vi "Change.vi"(6 "OldVal":variant, 8 "error in (no error)":errorcluster, 9 "NewVal":variant, 10 "Control Index":i32=-1, 11 "UndoObject in":refnum<class "UndoObject.lvclass">) -> (0 "error out":errorcluster, 1 "Redo Enable":bool, 2 "Undo Enable":bool, 3 "UndoObject out":refnum<class "UndoObject.lvclass">)   [LabVIEW 2015, in "UndoLibrary.lvlib" / "UndoObject.lvclass"]
doc: "This VI stores the changes produced in the controls. The maximum number of change is corresponding to the size of the buffer."
uses:
  UndoObject.lvclass
  UndoObject.lvclass/UndoObject.ctl
  Support VIs/DataClass/Controls/cluster_Control Value.ctl
  Support VIs/DataClass/DataObject.lvclass/DataObject.ctl
  <vilib>/Utility/error.llb/Error Cluster From Error Code.vi
  <vilib>/ErrorRing/Error Ring.xnode
  Support VIs/DataClass/DataObject.lvclass
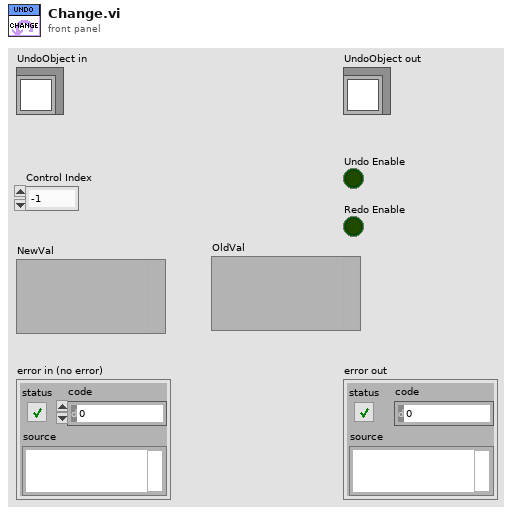
[diagram p1: front panel]
types:
  T1 = typedef "UndoLibrary.lvlib/DataObject.lvclass/cluster_Control Value.ctl" = cluster{"Index":i32, "Variant Data":variant}
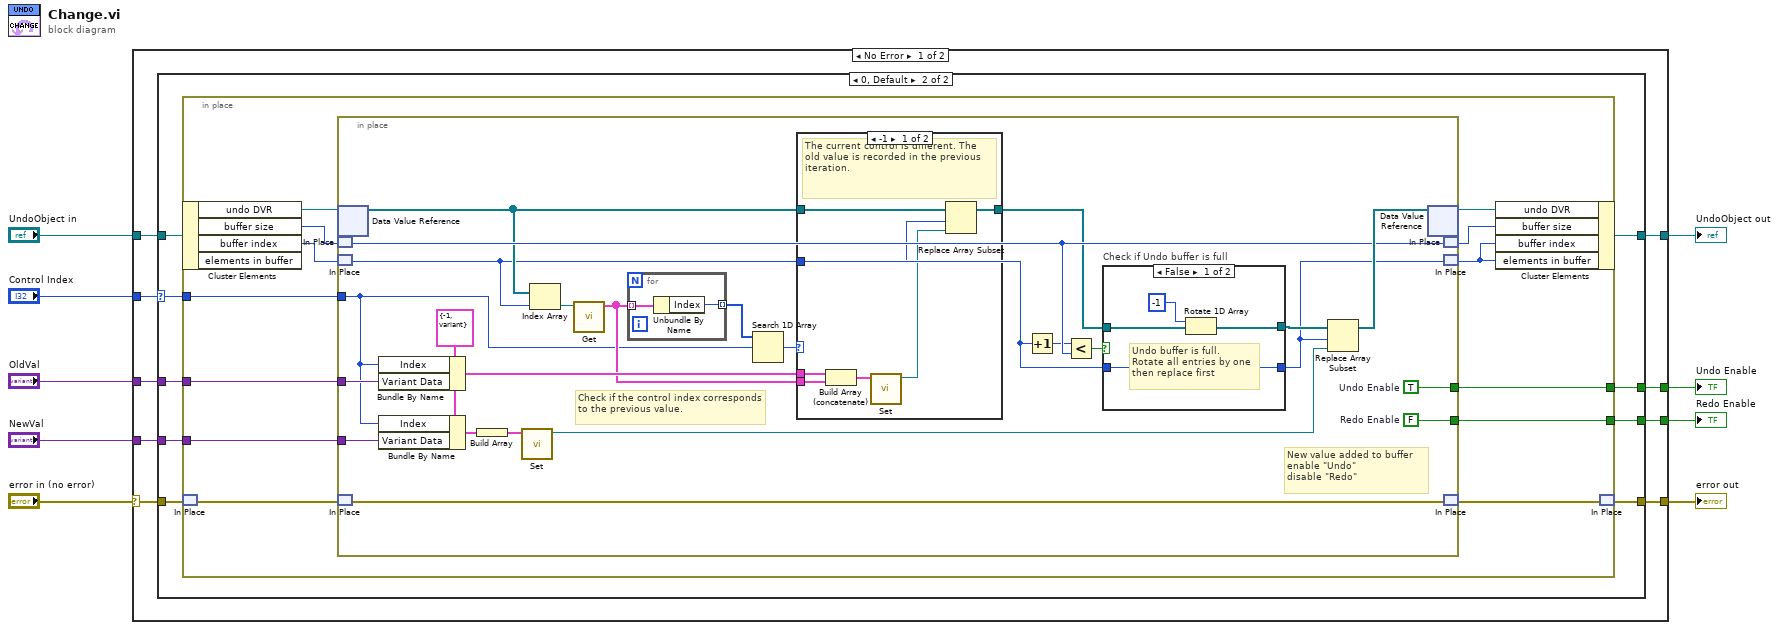
[diagram p0: block diagram]
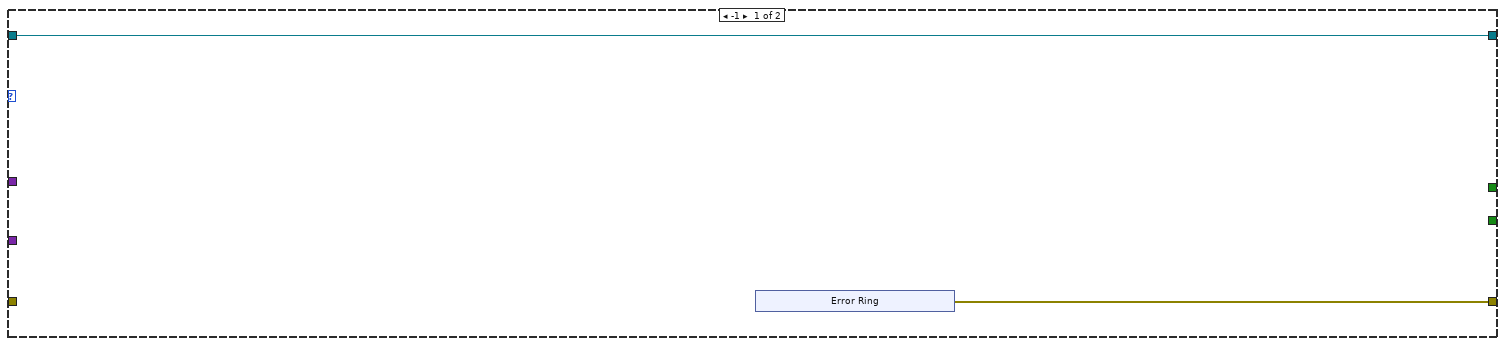
[diagram p2: hidden frame]
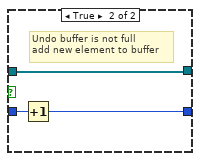
[diagram p4: hidden frame]
diagram:
  n1 = case shown="No Error" "error in (no error)" {
    selector: "error in (no error)" -> [w15 w89]
    tunnel: "OldVal" -> [w18 _]
    tunnel: "NewVal" -> [w17 _]
    tunnel: "Control Index" -> [w16 _]
    tunnel: "UndoObject in" -> [w13 w88]
    tunnel: [w12 w88] -> w2
    tunnel: [w14 w89] -> w5
    tunnel: [w11 _] -> w4
    tunnel: [w10 _] -> w1
    frame No Error {
      n2 = case shown="0, Default" w16 {
        selector: w16 -> [_ w31]
        tunnel: w18 -> [_ w33]
        tunnel: w17 -> [_ w32]
        tunnel: w15 -> [_ w29]
        tunnel: [w19 w28] -> w14
        tunnel: w13 -> [w20 w27]
        tunnel: [w20 w26] -> w12
        tunnel: [_ w30] -> w11
        tunnel: [_ w25] -> w10
        frame -1 {
          n3 = xnode "Error Ring"() -> ("error out"=w19:errorcluster)
        }
        frame 0, Default {
          n4 = in-place {
            in-place-border: w33 -> [w46]
            in-place-border: w32 -> [w45]
            in-place-border: w31 -> [w44]
            in-place-border: [w43] -> w30
            in-place-border: [w38] -> w25
            n5 = in-place-cluster #1(w27) -> ("undo DVR"=w40:refnum<data-value>, "buffer size"=w37:i32, "buffer index"=w35:i32)  [unwired: 1 out]
            n6 = in-place-match #2(w29) -> (w42:errorcluster)
            n7 = in-place {
              in-place-border: w46 -> [w69]
              in-place-border: w45 -> [w68]
              in-place-border: w44 -> [w48]
              in-place-border: [w66] -> w43
              in-place-border: [w60] -> w38
              w60 = TRUE  # Undo Enable
              w66 = FALSE  # Redo Enable
              w70 = T1 {"Index"=-1, "Variant Data"=variant} ("Control Value")
              # "Check if the control index corresponds to the previous value."
              # "New value added to buffer\nenable \"Undo\"\ndisable \"Redo\""
              n8 = in-place-dvr #3(w40) -> (w51:refnum<class "DataObject.lvclass">[])  [unwired: 1 out]
              n9 = in-place-match #4(w37) -> (w61:i32)
              n10 = in-place-match #5(w35) -> (w49:i32)
              n11 = in-place-match #6(w42) -> (w63:errorcluster)
              n12 = Bundle By Name(cluster=w70, "Index"=w48, "Variant Data"=w69) -> (w56:T1)
              n13 = Bundle By Name(cluster=w70, "Index"=w48, "Variant Data"=w68) -> (w67:T1)
              n14 = Build Array(w67) -> (w55:T1[])
              n15 = call "Set.vi"("Conrol Value[]"=w55) -> ("DataObject out"=w54:refnum<class "DataObject.lvclass">)  [unwired: 9 in, 1 out]
              n16 = Index Array(array=w51, index=w49) -> (element=w59:refnum<class "DataObject.lvclass">)
              n17 = call "Get.vi"("DataObject in"=w59) -> ("Conrol Value[]"=w52:T1[])  [unwired: 9 in, 1 out]
              n18 = for {
                tunnel: [w72] -> w57 mode=indexing
                tunnel: w52 -> [w71] mode=indexing
                n19 = Unbundle By Name(w71) -> ("Index"=w72:i32)
              }
              n20 = Search 1D Array(1D array=w57, element=w48) -> (index of element=w58:i32)  [unwired: 1 in]
              n21 = case shown="-1" w58 {
                tunnel: w56 -> [w79 _]
                tunnel: w52 -> [w77 _]
                tunnel: w51 -> [w76 w80]
                tunnel: [w75 w80] -> w50
                tunnel: w49 -> [w73 _]
                frame -1 {
                  # "The current control is different. The old value is recorded in the previous iteration."
                  n22 = Build Array (concatenate)(w79, w77) -> (w78:T1[])
                  n23 = call "Set.vi"("Conrol Value[]"=w78) -> ("DataObject out"=w74:refnum<class "DataObject.lvclass">)  [unwired: 9 in, 1 out]
                  n24 = Replace Array Subset(array=w76, new element=w74, index=w73) -> (w75:refnum<class "DataObject.lvclass">[])
                }
                frame 0, Default {
                  # "It is the same control."
                }
              }
              n25 = Increment(x=w49) -> (x+1=w53:i32)
              n26 = Less?(x=w53, y=w61) -> (x < y?=w62:bool)
              n27 = case "Check if Undo buffer is full" shown="False" w62 {
                tunnel: [w84 w87] -> w65
                tunnel: w49 -> [w81 w86]
                tunnel: w50 -> [w83 w87]
                tunnel: [w81 w85] -> w47
                frame False {
                  # "Undo buffer is full.\nRotate all entries by one\nthen replace first"
                  n28 = Rotate 1D Array(1:w83, 2:-1 ("n")) -> (0:w84:refnum<class "DataObject.lvclass">[])
                }
                frame True {
                  # "Undo buffer is not full\nadd new element to buffer"
                  n29 = Increment(x=w86) -> (x+1=w85:i32)
                }
              }
              n30 = Replace Array Subset(array=w65, new element=w54, index=w47) -> (w64:refnum<class "DataObject.lvclass">[])
              n31 = in-place-dvr #3(w64) -> (w39:refnum<data-value>)  [unwired: 1 out]
              n32 = in-place-match #4(w61) -> (w36:i32)
              n33 = in-place-match #5(w47) -> (w34:i32)
              n34 = in-place-match #6(w63) -> (w41:errorcluster)
            }
            n35 = in-place-cluster #1("undo DVR"=w39, "buffer size"=w36, "buffer index"=w34, "elements in buffer"=w34) -> (w26:refnum<class "UndoObject.lvclass">)
            n36 = in-place-match #2(w41) -> (w28:errorcluster)
          }
        }
      }
    }
    frame Error {
    }
  }
  "error out" <- w5
  "Undo Enable" <- w1
  "Redo Enable" <- w4
  "UndoObject out" <- w2
